vi "LINC Get Packet Info.vi"(8 "error in (no error)":errorcluster, 11 "packet":variant) -> (0 "error out":errorcluster, 1 "member data":string[](array[string]), 2 "member names":string[](array[string]), 3 "packet name":string, 5 "member types":string[](array[string]))   [LabVIEW 2018, in "STEPkgDriver_LINC.lvlib"]
uses:
  STEPkgDriver_LINC.lvlib
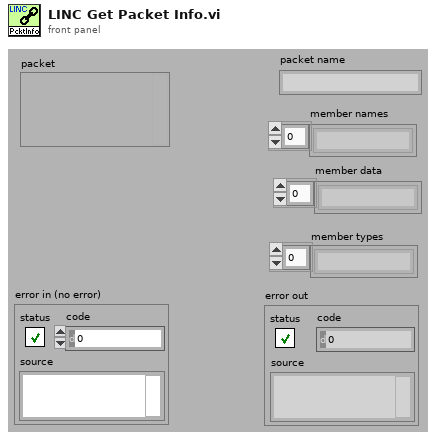
[diagram p1: front panel]
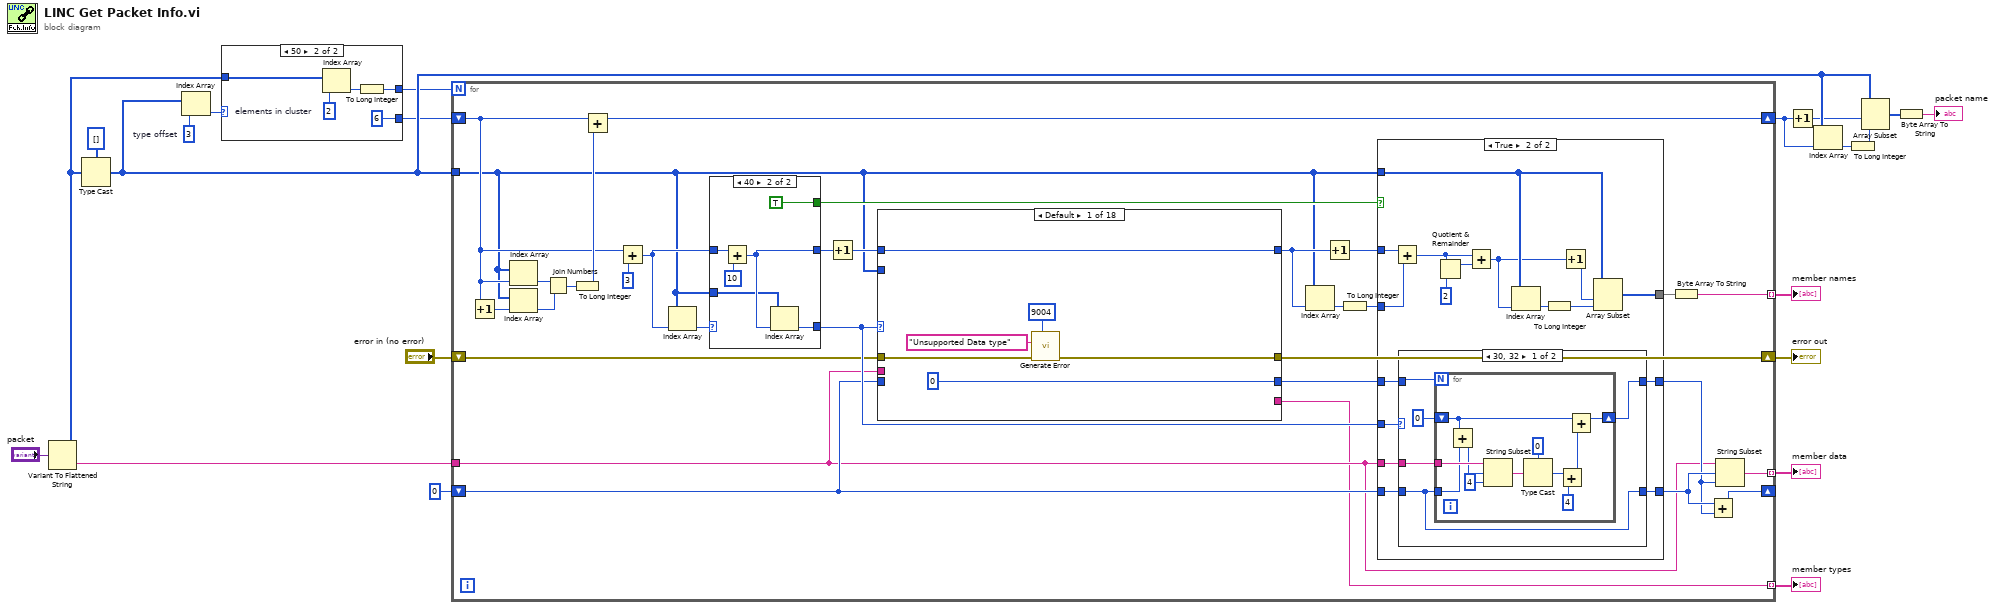
[diagram p0: block diagram]
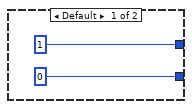
[diagram p2: hidden frame]
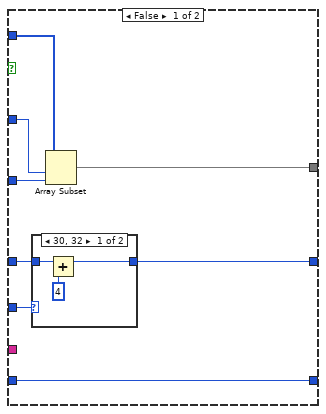
[diagram p3: hidden frame]
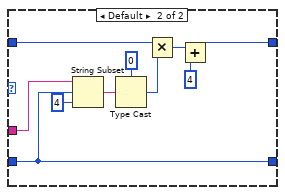
[diagram p5: hidden frame]
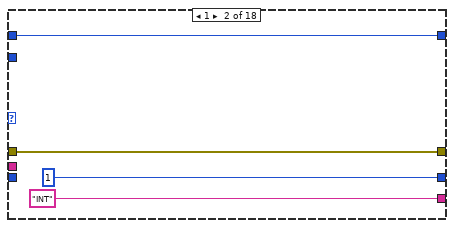
[diagram p7: hidden frame]
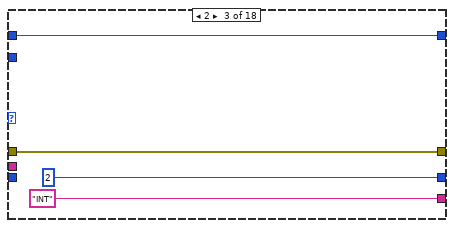
[diagram p8: hidden frame]
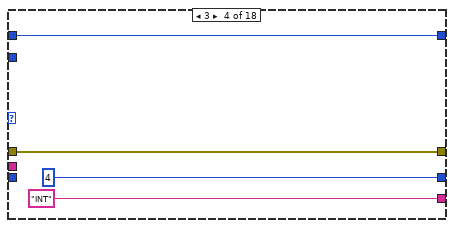
[diagram p9: hidden frame]
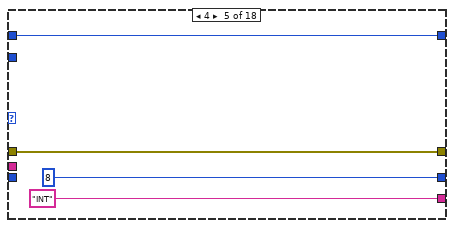
[diagram p10: hidden frame]
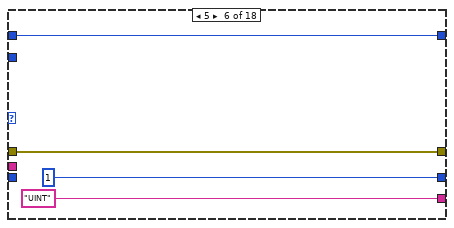
[diagram p11: hidden frame]
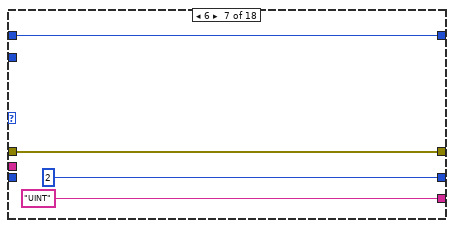
[diagram p12: hidden frame]
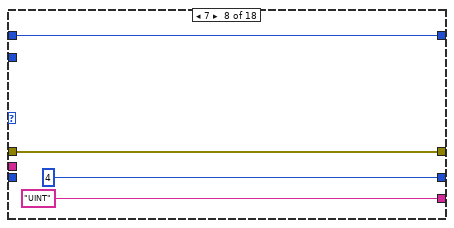
[diagram p13: hidden frame]
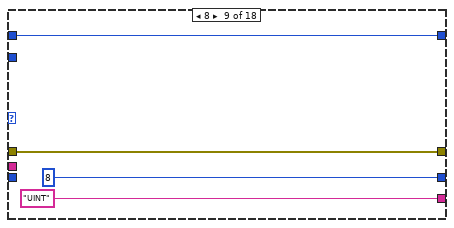
[diagram p14: hidden frame]
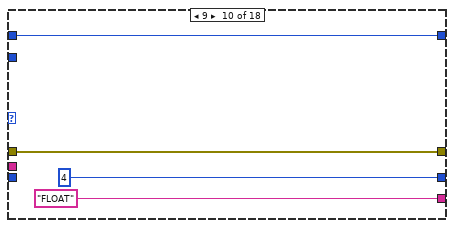
[diagram p15: hidden frame]
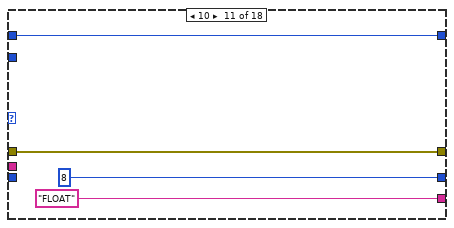
[diagram p16: hidden frame]
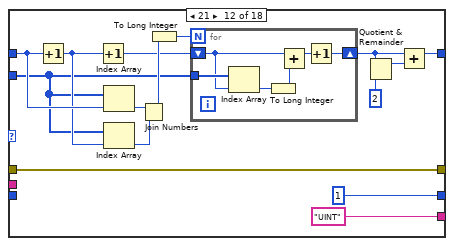
[diagram p17: hidden frame]
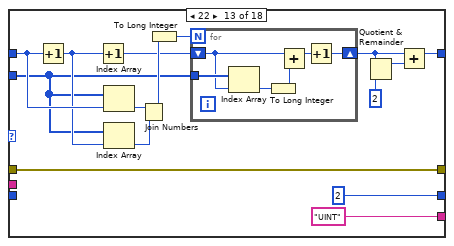
[diagram p18: hidden frame]
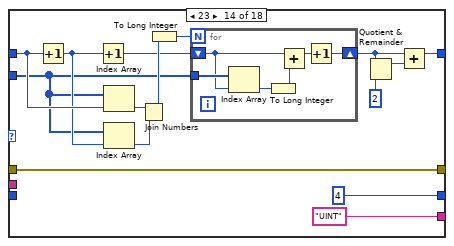
[diagram p19: hidden frame]
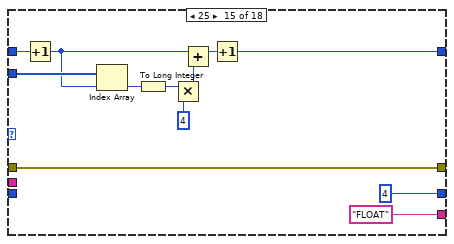
[diagram p20: hidden frame]
diagram:
  w19 = 3  # type offset
  n1 = Variant To Flattened String(Variant="packet") -> (data string=w21:string, 1:w16:i16[])
  n2 = Type Cast(type=u8[] [], x=w16) -> (*(type *) &x=w11:u8[])
  n3 = Index Array(array=w11, index=w19) -> (element=w1:u8)
  n4 = case shown="50" w1 {
    tunnel: w16 -> [_ w28]
    tunnel: [1 w25] -> w9
    tunnel: [0 6] -> w7
    frame Default {
    }
    frame 80 {
      w27 = 2  # elements in cluster
      n5 = Index Array(array=w28, index=w27) -> (element=w26:i16)
      n6 = To Long Integer(number=w26) -> (32bit integer=w25:i32)
    }
  }
  n7 = for {
    N: w9 -> [_]
    tunnel: w21 -> [w38]
    tunnel: w11 -> [w34]
    shift-right: [w48] -> w3
    shift-left: w7 -> [w35]
    tunnel: [w50] -> w18 mode=indexing
    shift-right: [w56] -> _
    shift-left: 0 -> [w39]
    tunnel: [w55] -> w17 mode=indexing
    shift-right: [w36] -> w13
    shift-left: "error in (no error)" -> [w37]
    tunnel: [w29] -> w10 mode=indexing
    n8 = Increment(x=w35) -> (x+1=w33:i32)
    n9 = Index Array(array=w34, index=w35) -> (element=w32:u8)
    n10 = Index Array(array=w34, index=w33) -> (element=w31:u8)
    n11 = Join Numbers(hi=w32, lo=w31) -> ((hi.lo)=w30:u16)
    n12 = To Long Integer(number=w30) -> (32bit integer=w49:i32)
    n13 = Add(x=w35, y=w49) -> (x+y=w48:i32)
    n14 = Add(x=w35, y=3) -> (x+y=w47:i32)
    n15 = Index Array(array=w34, index=w47) -> (element=w59:u8)
    n16 = case shown="40" w59 {
      selector: w59 -> [w116 _]
      tunnel: [w116 w122] -> w40
      tunnel: w34 -> [_ w117]
      tunnel: [_ TRUE] -> w44
      tunnel: w47 -> [w115 w120]
      tunnel: [w115 w118] -> w58
      frame Default {
      }
      frame 64 {
        n17 = Add(x=w120, y=10) -> (x+y=w118:i32)
        n18 = Index Array(array=w117, index=w118) -> (element=w122:u8)
      }
    }
    n19 = Increment(x=w58) -> (x+1=w57:i32)
    n20 = case shown="Default" w40 {
      tunnel: [0 ("size") 1 ("size") 2 ("size") 4 ("size") 8 ("size") 1 ("size") 2 ("size") 4 ("size") 8 ("size") 4 ("size") 8 ("size") 1 ("size") 2 ("size") 4 ("size") 4 ("size") 8 ("size") 1 ("size") w262] -> w42
      tunnel: w57 -> [w127 w131 w135 w139 w143 w147 w151 w155 w159 w163 w167 w182 w203 w224 w241 w253 w258 w269]
      tunnel: [w127 w131 w135 w139 w143 w147 w151 w155 w159 w163 w167 w172 w193 w214 w234 w246 w258 w268] -> w45
      tunnel: w34 -> [_ _ _ _ _ _ _ _ _ _ _ w176 w197 w218 w242 w254 _ _]
      tunnel: w38 -> [_ _ _ _ _ _ _ _ _ _ _ _ _ _ _ _ _ w267]
      tunnel: w39 -> [_ _ _ _ _ _ _ _ _ _ _ _ _ _ _ _ _ w263]
      tunnel: w37 -> [w125 w130 w134 w138 w142 w146 w150 w154 w158 w162 w166 w170 w191 w212 w233 w245 w257 w261]
      tunnel: [w123 w130 w134 w138 w142 w146 w150 w154 w158 w162 w166 w170 w191 w212 w233 w245 w257 w261] -> w36
      tunnel: [_ "INT" "INT" "INT" "INT" "UINT" "UINT" "UINT" "UINT" "FLOAT" "FLOAT" "UINT" "UINT" "UINT" "FLOAT" "FLOAT" "UINT" "STRING"] -> w29
      frame Default {
        n21 = call "Generate Error.vi"("error code (-1301)"=9004, "error in"=w125, "description"="Unsupported Data type") -> ("error out"=w123:errorcluster)  [unwired: 8 in]
      }
      frame 1 {
      }
      frame 2 {
      }
      frame 3 {
      }
      frame 4 {
      }
      frame 5 {
      }
      frame 6 {
      }
      frame 7 {
      }
      frame 8 {
      }
      frame 9 {
      }
      frame 10 {
      }
      frame 21 {
        n22 = Increment(x=w182) -> (x+1=w178:i32)
        n23 = Increment(x=w178) -> (x+1=w177:i32)
        n24 = Index Array(array=w176, index=w182) -> (element=w181:u8)
        n25 = Index Array(array=w176, index=w178) -> (element=w180:u8)
        n26 = Join Numbers(hi=w181, lo=w180) -> ((hi.lo)=w179:u16)
        n27 = To Long Integer(number=w179) -> (32bit integer=w171:i32)
        n28 = for {
          N: w171 -> [_]
          shift-right: [w186] -> w174
          shift-left: w177 -> [w188]
          tunnel: w176 -> [w189]
          n29 = Index Array(array=w189, index=w188) -> (element=w185:u8)
          n30 = To Long Integer(number=w185) -> (32bit integer=w184:i32)
          n31 = Add(x=w188, y=w184) -> (x+y=w187:i32)
          n32 = Increment(x=w187) -> (x+1=w186:i32)
        }
        n33 = Quotient & Remainder(x=w174, y=2) -> (x-y*floor(x/y)=w173:i32)  [unwired: 1 out]
        n34 = Add(x=w174, y=w173) -> (x+y=w172:i32)
      }
      frame 22 {
        n35 = Increment(x=w203) -> (x+1=w199:i32)
        n36 = Increment(x=w199) -> (x+1=w198:i32)
        n37 = Index Array(array=w197, index=w203) -> (element=w202:u8)
        n38 = Index Array(array=w197, index=w199) -> (element=w201:u8)
        n39 = Join Numbers(hi=w202, lo=w201) -> ((hi.lo)=w200:u16)
        n40 = To Long Integer(number=w200) -> (32bit integer=w192:i32)
        n41 = for {
          N: w192 -> [_]
          shift-right: [w207] -> w195
          shift-left: w198 -> [w209]
          tunnel: w197 -> [w210]
          n42 = Index Array(array=w210, index=w209) -> (element=w206:u8)
          n43 = To Long Integer(number=w206) -> (32bit integer=w205:i32)
          n44 = Add(x=w209, y=w205) -> (x+y=w208:i32)
          n45 = Increment(x=w208) -> (x+1=w207:i32)
        }
        n46 = Quotient & Remainder(x=w195, y=2) -> (x-y*floor(x/y)=w194:i32)  [unwired: 1 out]
        n47 = Add(x=w195, y=w194) -> (x+y=w193:i32)
      }
      frame 23 {
        n48 = Increment(x=w224) -> (x+1=w220:i32)
        n49 = Increment(x=w220) -> (x+1=w219:i32)
        n50 = Index Array(array=w218, index=w224) -> (element=w223:u8)
        n51 = Index Array(array=w218, index=w220) -> (element=w222:u8)
        n52 = Join Numbers(hi=w223, lo=w222) -> ((hi.lo)=w221:u16)
        n53 = To Long Integer(number=w221) -> (32bit integer=w213:i32)
        n54 = for {
          N: w213 -> [_]
          shift-right: [w228] -> w216
          shift-left: w219 -> [w230]
          tunnel: w218 -> [w231]
          n55 = Index Array(array=w231, index=w230) -> (element=w227:u8)
          n56 = To Long Integer(number=w227) -> (32bit integer=w226:i32)
          n57 = Add(x=w230, y=w226) -> (x+y=w229:i32)
          n58 = Increment(x=w229) -> (x+1=w228:i32)
        }
        n59 = Quotient & Remainder(x=w216, y=2) -> (x-y*floor(x/y)=w215:i32)  [unwired: 1 out]
        n60 = Add(x=w216, y=w215) -> (x+y=w214:i32)
      }
      frame 25 {
        n61 = Increment(x=w241) -> (x+1=w237:i32)
        n62 = Index Array(array=w242, index=w237) -> (element=w240:u8)
        n63 = To Long Integer(number=w240) -> (32bit integer=w239:i32)
        n64 = Multiply(x=w239, y=4) -> (x*y=w236:i32)
        n65 = Add(x=w237, y=w236) -> (x+y=w235:i32)
        n66 = Increment(x=w235) -> (x+1=w234:i32)
      }
      frame 26 {
        n67 = Increment(x=w253) -> (x+1=w249:i32)
        n68 = Index Array(array=w254, index=w249) -> (element=w252:u8)
        n69 = To Long Integer(number=w252) -> (32bit integer=w251:i32)
        n70 = Multiply(x=w251, y=4) -> (x*y=w248:i32)
        n71 = Add(x=w249, y=w248) -> (x+y=w247:i32)
        n72 = Increment(x=w247) -> (x+1=w246:i32)
      }
      frame 33 {
      }
      frame 48, 50 {
        n73 = Add(x=w269, y=4) -> (x+y=w268:i32)
        n74 = String Subset(string=w267, offset (0)=w263, length (rest)=4 ("length (rest)")) -> (substring=w265:string)
        n75 = Type Cast(type=0, x=w265) -> (*(type *) &x=w262:i32)
      }
    }
    n76 = Index Array(array=w34, index=w45) -> (element=w53:u8)
    n77 = Increment(x=w45) -> (x+1=w51:i32)
    n78 = To Long Integer(number=w53) -> (32bit integer=w52:i32)
    n79 = case shown="True" w44 {
      tunnel: [w67 w88] -> w54
      tunnel: w52 -> [w63 w87]
      tunnel: w51 -> [w66 w78]
      tunnel: w34 -> [w65 w86]
      tunnel: w38 -> [_ w79]
      tunnel: w39 -> [w64 w83]
      tunnel: [w64 w82] -> w43
      tunnel: w42 -> [w61 w81]
      tunnel: [w60 w80] -> w41
      tunnel: w40 -> [w62 w72]
      frame False {
        n80 = case shown="30, 32" w62 {
          tunnel: w61 -> [w69 w71]
          tunnel: [w68 w71] -> w60
          frame 48, 50 {
            n81 = Add(x=w69, y=4) -> (x+y=w68:i32)
          }
          frame Default {
          }
        }
        n82 = Array Subset(array=w65, index=w66, length=w63) -> (w67:u8[])
      }
      frame True {
        n83 = Add(x=w78, y=w87) -> (x+y=w74:i32)
        n84 = case shown="30, 32" w72 {
          tunnel: w83 -> [w89 w108]
          tunnel: [w89 w108] -> w82
          tunnel: w81 -> [w93 w111]
          tunnel: [w90 w105] -> w80
          tunnel: w79 -> [w92 w109]
          frame 48, 50 {
            n85 = for {
              N: w93 -> [_]
              tunnel: w92 -> [w101]
              shift-right: [w100] -> w90
              shift-left: 0 -> [w96]
              tunnel: w89 -> [w95]
              n86 = Add(x=w96, y=w95) -> (x+y=w94:i32)
              n87 = String Subset(string=w101, offset (0)=w94, length (rest)=4 ("length (rest)")) -> (substring=w103:string)
              n88 = Type Cast(type=0, x=w103) -> (*(type *) &x=w98:i32)
              n89 = Add(x=w98, y=4) -> (x+y=w97:i32)
              n90 = Add(x=w96, y=w97) -> (x+y=w100:i32)
            }
          }
          frame Default {
            n91 = String Subset(string=w109, offset (0)=w108, length (rest)=4 ("length (rest)")) -> (substring=w113:string)
            n92 = Type Cast(type=0, x=w113) -> (*(type *) &x=w110:i32)
            n93 = Multiply(x=w111, y=w110) -> (x*y=w106:i32)
            n94 = Add(x=w106, y=4) -> (x+y=w105:i32)
          }
        }
        n95 = Quotient & Remainder(x=w74, y=2) -> (x-y*floor(x/y)=w75:i32)  [unwired: 1 out]
        n96 = Add(x=w74, y=w75) -> (x+y=w73:i32)
        n97 = Index Array(array=w86, index=w73) -> (element=w84:u8)
        n98 = To Long Integer(number=w84) -> (32bit integer=w77:i32)
        n99 = Increment(x=w73) -> (x+1=w85:i32)
        n100 = Array Subset(array=w86, index=w85, length=w77) -> (w88:u8[])
      }
    }
    n101 = Byte Array To String(unsigned byte array=w54) -> (string=w50:string)
    n102 = Add(x=w43, y=w41) -> (x+y=w56:i32)
    n103 = String Subset(string=w38, offset (0)=w43, length (rest)=w41) -> (substring=w55:string)
  }
  "member names" <- w18
  "member data" <- w17
  "error out" <- w13
  "member types" <- w10
  n104 = Increment(x=w3) -> (x+1=w2:i32)
  n105 = Index Array(array=w11, index=w3) -> (element=w6:u8)
  n106 = To Long Integer(number=w6) -> (32bit integer=w4:i32)
  n107 = Array Subset(array=w11, index=w2, length=w4) -> (w5:u8[])
  n108 = Byte Array To String(unsigned byte array=w5) -> (string=→"packet name":string)
